vi "Execute.vi"(8 "error in (no error)":errorcluster, 10 "Context in":refnum<class "Context.lvclass">, 11 "Start Scan Command in":refnum<class "Complete Testing Command.lvclass">) -> (0 "error out":errorcluster, 2 "Context out":refnum<class "Context.lvclass">, 3 "Start Scan Command out":refnum<class "Complete Testing Command.lvclass">)   [LabVIEW 2015, in "Complete Testing Command.lvclass"]
uses:
  Complete Testing Command.lvclass
  Context/Context.lvclass
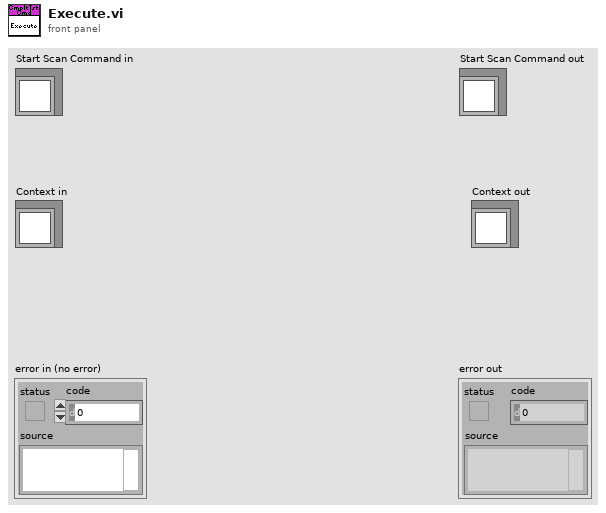
[diagram p1: front panel]
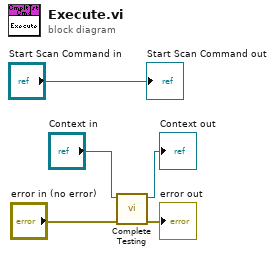
[diagram p0: block diagram]
diagram:
  n1 = call "Complete Testing.vi"("error in (no error)"="error in (no error)", "Context in"="Context in") -> ("error out"=→"error out":errorcluster, "Context out"=→"Context out":refnum<class "Context.lvclass">)  [unwired: 8 in]
  "Start Scan Command out" <- "Start Scan Command in"
